vi "SetSlitwidth.vi"(8 "error in (no error)":errorcluster, 9 "Slitwidth":u16, 10 "Slit":T1, 11 "DongWoo in":refnum<class "DongWoo.lvclass">) -> (0 "error out":errorcluster, 3 "DongWoo out":refnum<class "DongWoo.lvclass">)   [LabVIEW 2023, in "DongWoo_Spectrometer.lvlib" / "DongWoo.lvclass"]
uses:
  typedefs/SpectrSlitControl.ctl
  DongWoo.lvclass
  DongWoo.lvclass/DongWoo.ctl
  typedefs/typedefs.lvlib
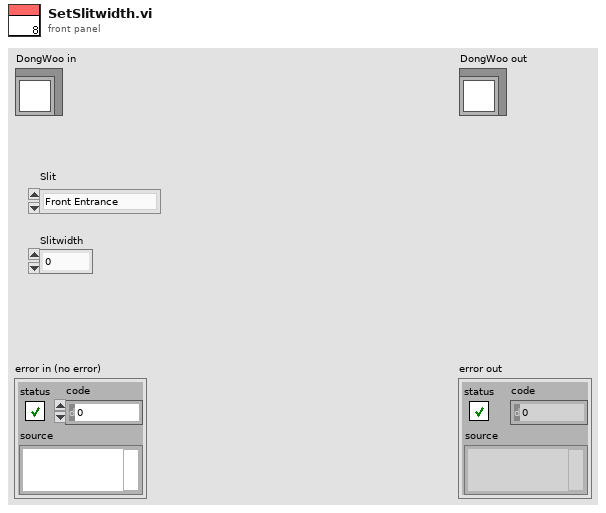
[diagram p1: front panel]
types:
  T1 = typedef "typedefs.lvlib/SpectrSlitControl.ctl" = enum16{"Front Entrance", "Side Entrance", "Front Exit", "Side Exit"}
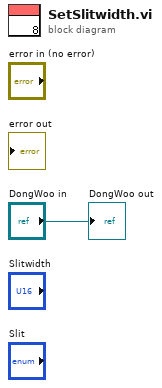
[diagram p0: block diagram]
diagram:
  "DongWoo out" <- "DongWoo in"
